vi "Bundle.vi"(6 "Restore Range if Changed?(T)":bool=TRUE, 7 "Check Range?(T)":bool=TRUE, 8 "error in (no error)":errorcluster, 9 "Max Time(-1ms)":i32=-1, 10 "Measurements to Acquire(1)":i32=1, 11 "DMM Triggered Measure Msg in":refnum<class "DMM Triggered Measure Msg.lvclass">) -> (0 "error out":errorcluster, 3 "DMM Triggered Measure Msg out":refnum<class "DMM Triggered Measure Msg.lvclass">)   [LabVIEW 2020, in "DMM Msg.lvlib" / "DMM Triggered Measure Msg.lvclass"]
doc: "Populate the message."
uses:
  DMM Triggered Measure Msg.lvclass
  DMM Triggered Measure Msg.lvclass/DMM Triggered Measure Msg.ctl
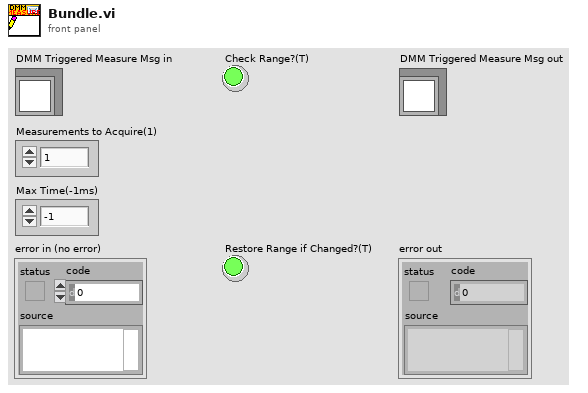
[diagram p1: front panel]
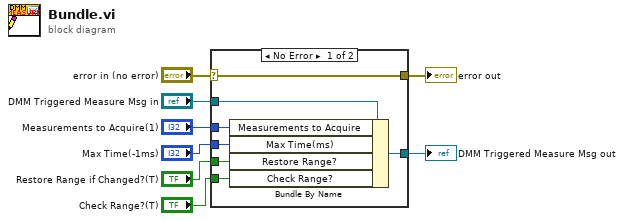
[diagram p0: block diagram]
diagram:
  n1 = case shown="No Error" "error in (no error)" {
    selector: "error in (no error)" -> [w15 w16]
    tunnel: [w15 w16] -> w7
    tunnel: [w13 w17] -> w5
    tunnel: "DMM Triggered Measure Msg in" -> [w14 w17]
    tunnel: "Measurements to Acquire(1)" -> [w12 _]
    tunnel: "Max Time(-1ms)" -> [w11 _]
    tunnel: "Restore Range if Changed?(T)" -> [w10 _]
    tunnel: "Check Range?(T)" -> [w9 _]
    frame No Error {
      n2 = Bundle By Name(cluster=w14, "Measurements to Acquire"=w12, "Max Time(ms)"=w11, "Restore Range?"=w10, "Check Range?"=w9) -> (w13:refnum<class "DMM Triggered Measure Msg.lvclass">)
    }
    frame Error {
    }
  }
  "error out" <- w7
  "DMM Triggered Measure Msg out" <- w5
